vi "CANOpen_Check_Node_State for Node without HB NG.vi"(7 "State detect in None":T1=enum."HB", 8 "error in":errorcluster, 9 "Node ID":u8, 11 "interface object in":refnum<k20>) -> (0 "error out":errorcluster, 1 "Last State":u16, 2 "Time for read":u32, 4 "timestamp":timestamp)   [LabVIEW 2013, in "CANOpen Addon Custom Device.lvlib"]
uses:
  CANOpen Addon Custom Device.lvlib
  CanOpen_NMT_Static detect.ctl
  <vilib>/CANopenLib/CANOPEN.llb/CANopen SDO Create.vi
  <vilib>/CANopenLib/CANOPEN.llb/CANopen SDO Write [U16].vi
  <vilib>/CANopenLib/CANOPEN.llb/CANopen SDO Write [U8].vi
  <vilib>/CANopenLib/CANOPEN.llb/CANopen Node Guarding Create.vi
  <vilib>/CANopenLib/CANOPEN.llb/CANopen Node Guarding Start.vi
  <vilib>/CANopenLib/CANOPEN.llb/CANopen Node Guarding State Read.vi
  <vilib>/CANopenLib/CANOPEN.llb/CANopen SDO Close.vi
  <vilib>/CANopenLib/CANOPEN.llb/CANopen Node Guarding Stop.vi
  <vilib>/CANopenLib/CANOPEN.llb/CANopen Node Guarding Close.vi
  <vilib>/CANopenLib/CANOPEN.llb/CANopen Heartbeat Create.vi
  <vilib>/CANopenLib/CANOPEN.llb/CANopen Heartbeat Start.vi
  <vilib>/CANopenLib/CANOPEN.llb/CANopen Heartbeat State Read.vi
  <vilib>/CANopenLib/CANOPEN.llb/CANopen Heartbeat Stop.vi
  <vilib>/CANopenLib/CANOPEN.llb/CANopen Heartbeat Close.vi
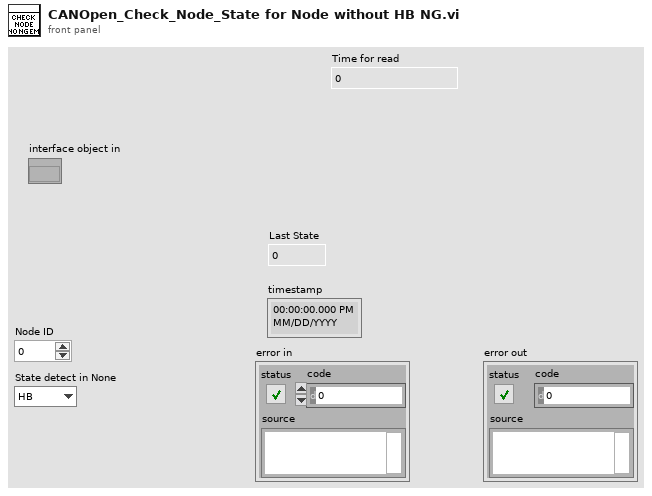
[diagram p1: front panel]
types:
  T1 = typedef "CANOpen Addon Custom Device.lvlib/CanOpen_NMT_Static detect.ctl" = enum16{"None", "HB", "NG"}
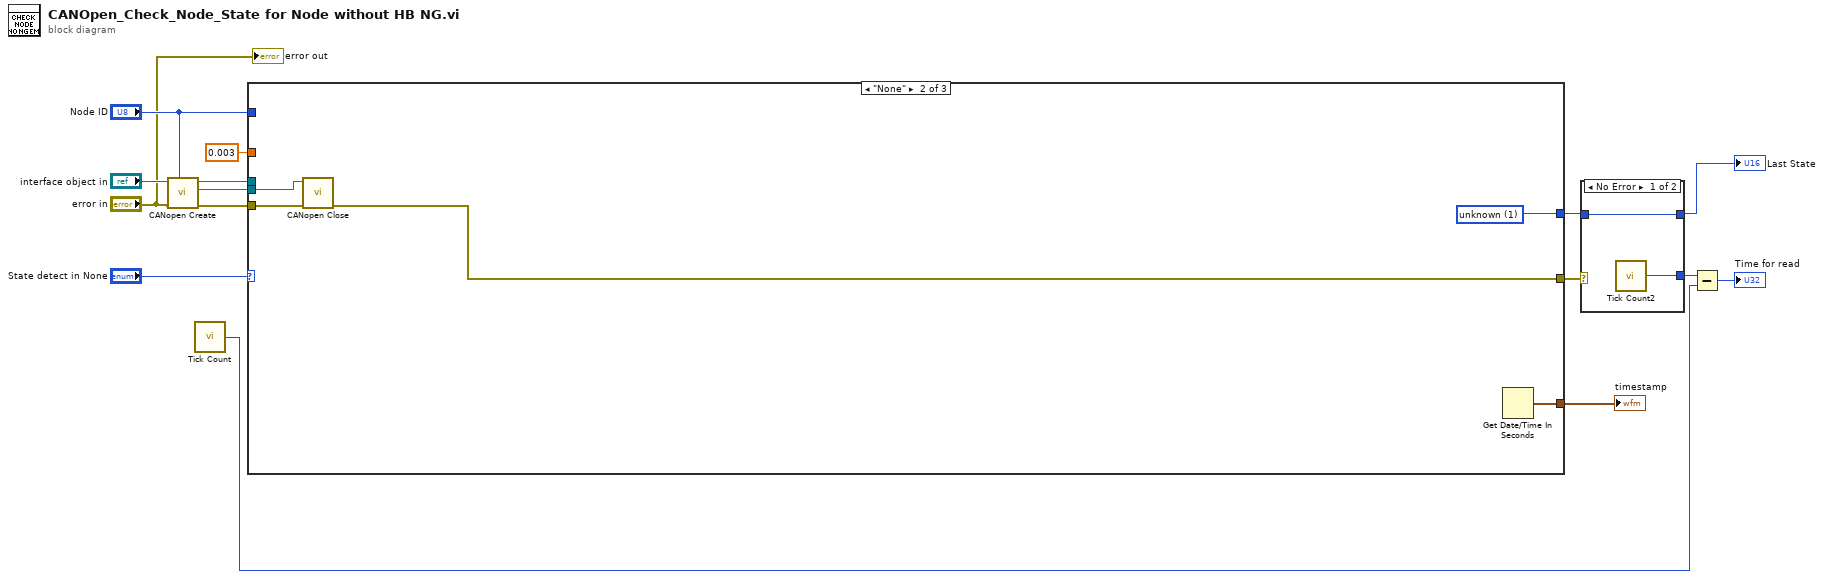
[diagram p0: block diagram]
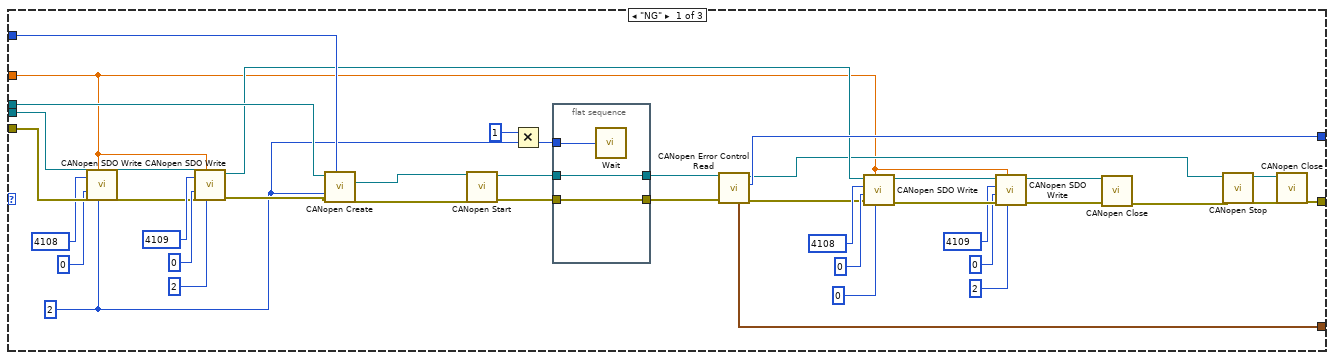
[diagram p2: hidden frame]
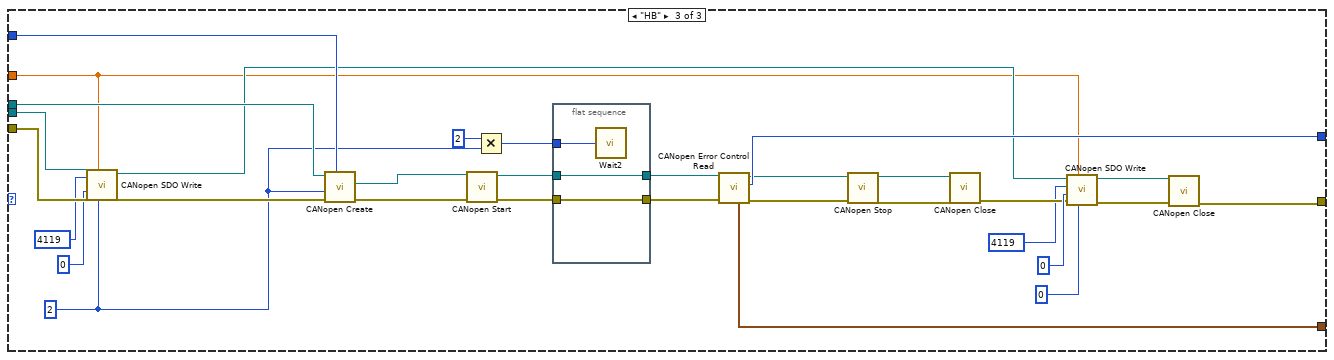
[diagram p3: hidden frame]
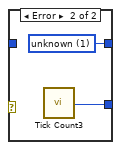
[diagram p4: hidden frame]
diagram:
  n1 = call-poly <vilib>:"CANopen Create.vi"("node-ID"="Node ID", "error in (no error)"="error in", "interface object in"="interface object in") -> ("error out"=w9:errorcluster, "SDO object out"=w10:refnum<k20>, "interface object out"=w8:refnum<k20>)  [unwired: 6 in]
  n2 = call "Tick Count"() -> ("Tick Count(mSec)"=w3:u32)
  n3 = case shown="\"None\"" "State detect in None" {
    tunnel: [w52 w64 w91] -> w15
    tunnel: [w51 w61 w70] -> w13
    tunnel: [w50 w63 w90] -> w12
    tunnel: "Node ID" -> [w47 _ w87]
    tunnel: w10 -> [w46 w60 w86]
    tunnel: w9 -> [w45 w62 w85]
    tunnel: w8 -> [w42 _ w83]
    tunnel: 0.003 ("timeout (1s)") -> [w16 _ w65]
    frame "NG" {
      w19 = u16 2 ("Guard Time (ms)")
      n4 = call-poly <vilib>:"CANopen SDO Write.vi"("U16 data"=w19, "timeout (1s)"=w16, "error in (no error)"=w45, "object sub-index (0)"=u8 0, "object index"=u16 4108, "SDO object in"=w46) -> ("error out"=w38:errorcluster, "SDO object out"=w39:refnum<k20>)  [unwired: 3 in, 1 out]
      n5 = call-poly <vilib>:"CANopen SDO Write.vi"("U8 data"=u8 2, "timeout (1s)"=w16, "error in (no error)"=w38, "object sub-index (0)"=u8 0, "object index"=u16 4109, "SDO object in"=w39) -> ("error out"=w23:errorcluster, "SDO object out"=w22:refnum<k20>)  [unwired: 3 in, 1 out]
      n6 = call-poly <vilib>:"CANopen Create.vi"("node-ID"=w47, "error in (no error)"=w23, "guard time [ms]"=w19, "interface object in"=w42) -> ("error out"=w36:errorcluster, "node guarding object out"=w35:refnum<k20>)  [unwired: 5 in, 1 out]
      n7 = call-poly <vilib>:"CANopen Start.vi"("error in (no error)"=w36, "node guarding object in"=w35) -> ("error out"=w53:errorcluster, "node guarding object out"=w54:refnum<k20>)  [unwired: 8 in]
      n8 = Multiply(x=u16 1, y=w19) -> (x*y=w18:u16)
      n9 = flat-sequence {
        tunnel: w53 -> [w59]
        tunnel: w54 -> [w58]
        tunnel: [w59] -> w55
        tunnel: [w58] -> w56
        tunnel: w18 -> [w57]
        frame #0 {
          n10 = call "Wait"("Count(mSec)"=w57) -> ()  [unwired: 1 out]
        }
      }
      n11 = call-poly <vilib>:"CANopen Error Control Read.vi"("error in (no error)"=w55, "node guarding object in"=w56) -> ("error out"=w24:errorcluster, "state"=w52:u16, "node guarding object out"=w20:refnum<k20>, "timestamp"=w50:timestamp)  [unwired: 6 in]
      n12 = call-poly <vilib>:"CANopen SDO Write.vi"("U16 data"=u16 0, "timeout (1s)"=w16, "error in (no error)"=w24, "object sub-index (0)"=u8 0, "object index"=u16 4108, "SDO object in"=w22) -> ("error out"=w33:errorcluster, "SDO object out"=w32:refnum<k20>)  [unwired: 3 in, 1 out]
      n13 = call-poly <vilib>:"CANopen SDO Write.vi"("U8 data"=u8 2, "timeout (1s)"=w16, "error in (no error)"=w33, "object sub-index (0)"=u8 0, "object index"=u16 4109, "SDO object in"=w32) -> ("error out"=w27:errorcluster, "SDO object out"=w25:refnum<k20>)  [unwired: 3 in, 1 out]
      n14 = call-poly <vilib>:"CANopen Close.vi"("error in (no error)"=w27, "SDO object in"=w25) -> ("error out"=w21:errorcluster)  [unwired: 9 in]
      n15 = call-poly <vilib>:"CANopen Stop.vi"("error in (no error)"=w21, "node guarding object in"=w20) -> ("error out"=w49:errorcluster, "node guarding object out"=w48:refnum<k20>)  [unwired: 8 in]
      n16 = call-poly <vilib>:"CANopen Close.vi"("error in (no error)"=w49, "node guarding object in"=w48) -> ("error out"=w51:errorcluster)  [unwired: 9 in]
    }
    frame "None" {
      w64 = u16 1 items=["unknown"=1, "bootup"=0, "stopped"=4, "operational"=5, "pre-operational"=127, "connection lost"=128] ("State 2")
      n17 = call-poly <vilib>:"CANopen Close.vi"("error in (no error)"=w62, "SDO object in"=w60) -> ("error out"=w61:errorcluster)  [unwired: 9 in]
      n18 = Get Date/Time In Seconds() -> (seconds since 1Jan1904=w63:timestamp)
    }
    frame "HB" {
      w67 = u16 2 ("Guard Time (ms)")
      n19 = call-poly <vilib>:"CANopen SDO Write.vi"("U16 data"=w67, "timeout (1s)"=w65, "error in (no error)"=w85, "object sub-index (0)"=u8 0, "object index"=u16 4119, "SDO object in"=w86) -> ("error out"=w79:errorcluster, "SDO object out"=w69:refnum<k20>)  [unwired: 3 in, 1 out]
      n20 = call-poly <vilib>:"CANopen Create.vi"("node-ID"=w87, "error in (no error)"=w79, "consumer time [ms]"=w67, "interface object in"=w83) -> ("error out"=w82:errorcluster, "heartbeat object out"=w78:refnum<k20>)  [unwired: 5 in, 1 out]
      n21 = call-poly <vilib>:"CANopen Start.vi"("error in (no error)"=w82, "heartbeat object in"=w78) -> ("error out"=w92:errorcluster, "heartbeat object out"=w93:refnum<k20>)  [unwired: 8 in]
      n22 = Multiply(x=u16 2, y=w67) -> (x*y=w68:u16)
      n23 = flat-sequence {
        tunnel: w92 -> [w98]
        tunnel: w93 -> [w97]
        tunnel: [w98] -> w94
        tunnel: [w97] -> w95
        tunnel: w68 -> [w96]
        frame #0 {
          n24 = call "Wait2"("Count(mSec)"=w96) -> ()  [unwired: 1 out]
        }
      }
      n25 = call-poly <vilib>:"CANopen Error Control Read.vi"("error in (no error)"=w94, "heartbeat object in"=w95) -> ("error out"=w77:errorcluster, "state"=w91:u16, "heartbeat object out"=w81:refnum<k20>, "timestamp"=w90:timestamp)  [unwired: 6 in]
      n26 = call-poly <vilib>:"CANopen Stop.vi"("error in (no error)"=w77, "heartbeat object in"=w81) -> ("error out"=w89:errorcluster, "heartbeat object out"=w88:refnum<k20>)  [unwired: 8 in]
      n27 = call-poly <vilib>:"CANopen Close.vi"("error in (no error)"=w89, "heartbeat object in"=w88) -> ("error out"=w72:errorcluster)  [unwired: 9 in]
      n28 = call-poly <vilib>:"CANopen SDO Write.vi"("U16 data"=u16 0, "timeout (1s)"=w65, "error in (no error)"=w72, "object sub-index (0)"=u8 0, "object index"=u16 4119, "SDO object in"=w69) -> ("error out"=w73:errorcluster, "SDO object out"=w74:refnum<k20>)  [unwired: 3 in, 1 out]
      n29 = call-poly <vilib>:"CANopen Close.vi"("error in (no error)"=w73, "SDO object in"=w74) -> ("error out"=w70:errorcluster)  [unwired: 9 in]
    }
  }
  "timestamp" <- w12
  n30 = case shown="No Error" w13 {
    tunnel: [w100 w102] -> w14
    tunnel: w15 -> [w100 _]
    tunnel: [w99 w101] -> w4
    frame No Error {
      n31 = call "Tick Count2"() -> ("Tick Count(mSec)"=w99:u32)
    }
    frame Error {
      w102 = u16 1 items=["unknown"=1, "bootup"=0, "stopped"=4, "operational"=5, "pre-operational"=127, "connection lost"=128] ("State 2")
      n32 = call "Tick Count3"() -> ("Tick Count(mSec)"=w101:u32)
    }
  }
  "Last State" <- w14
  n33 = Subtract(x=w4, y=w3) -> (x-y=→"Time for read":u32)
  "error out" <- "error in"
